vi "LS Acquisition Main (FPGA).vi"() -> ()   [LabVIEW 2013]
uses:
  <vilib>/rvi/Emulation/niFpgaSctlEmulationGetInTimedLoop.vi
  <vilib>/rvi/Emulation/niFpgaEmulationReportErrorSimple.vi
  <vilib>/rvi/Emulation/niFpgaGetClockAttributes.vi
  <vilib>/rvi/eio/common/nirviEmuTemplateMethod_errors.vi
  <vilib>/rvi/Emulation/niFpgaCriticalErrorInLSC.vi
  <vilib>/rvi/DataTransferAndStorage/Container/Common/niFpgaContainerExecOnDevCompGetState.vi
  <vilib>/rvi/FIFO/Fifo_Resource/nirvififoEmulationWriteFpgaImpl.vi
  <vilib>/rvi/DataTransferAndStorage/Container/Common/niFpgaContainerGetUniqueNameForEmu.vi
  <vilib>/rvi/interface/RandomDataEmulation/nirviRandomDataFPGAFIFO.vi
  <vilib>/rvi/interface/RandomDataEmulation/niFpgaRandomDataHandleErrors.vi
  <vilib>/rvi/eio/common/nirviEmuReportErrorAndStop.vi
  <vilib>/eio/EIONode/EIONode.xnode
  <vilib>/rvi/FXPMathLib/FxpAdd/XNode/nifxpmath_Add.xnode
  <vilib>/rvi/DataTransferAndStorage/Container/XNode/niFpgaContainer.xnode
  <vilib>/rvi/FIFO/Fifo_Resource/niFpgaFifoEmulationRefIn.vi
  <vilib>/rvi/FXPMathLib/sim/FxpSim.dll
panel:
  in  "B2offset":fxp<+/-,24,5>
  in  "B1offset":fxp<+/-,24,5>
  out "Anomaly Resamples":fxp<+/-,28,17>[](array[numeric])
  out "Bank2Active":bool
  out "Bank1Active":bool
  out "Bank2On":bool
  out "Bank1On":bool
  in  "Enable Readings":bool[](array[boolean])=[FALSE, FALSE, FALSE, FALSE, FALSE, FALSE, FALSE, FALSE, FALSE, FALSE, FALSE, FALSE]
  in  "Opens Resets":bool[](array[boolean])=[FALSE, FALSE, FALSE, FALSE, FALSE, FALSE, FALSE, FALSE, FALSE, FALSE]
  in  "Enable Opens":bool[](array[boolean])=[FALSE, FALSE, FALSE, FALSE, FALSE, FALSE, FALSE, FALSE, FALSE, FALSE]
  out "Opens Detected":u16[](array[numeric])
  out "Opens Loop Time (usec)":u32=1000
  in  "Bank2(Pulse/Const)":bool
  in  "Bank2Const(On/Off)":bool
  out "Cycle Starts":bool[](array[boolean])
  out "Cycles":u32[](array[numeric])
  in  "Bank1Const(On/Off)":bool
  in  "Bank1(Pulse/Const)":bool
  in  "PWM Period (Ticks)":u32=4000000
  in  "Duty (Ticks)":i32=2000000
  in  "Invert PWM?":bool=TRUE
  in  "Cycle Resets":bool[](array[boolean])=[FALSE, FALSE, FALSE, FALSE, FALSE, FALSE, FALSE, FALSE, FALSE, FALSE]
  in  "Points to Avg":i32=20
  in  "Enable Cycles":bool[](array[boolean])=[FALSE, FALSE, FALSE, FALSE, FALSE, FALSE, FALSE, FALSE, FALSE, FALSE]
  out "Total Cycles":u32[](array[numeric])
  in  "Cycle Threshold":fxp<+/-,28,17>=1.2001953125
  out "Analog Inputs":fxp<+/-,28,17>[](array[numeric])
  out "AI Loop Time (usec)":u32=70
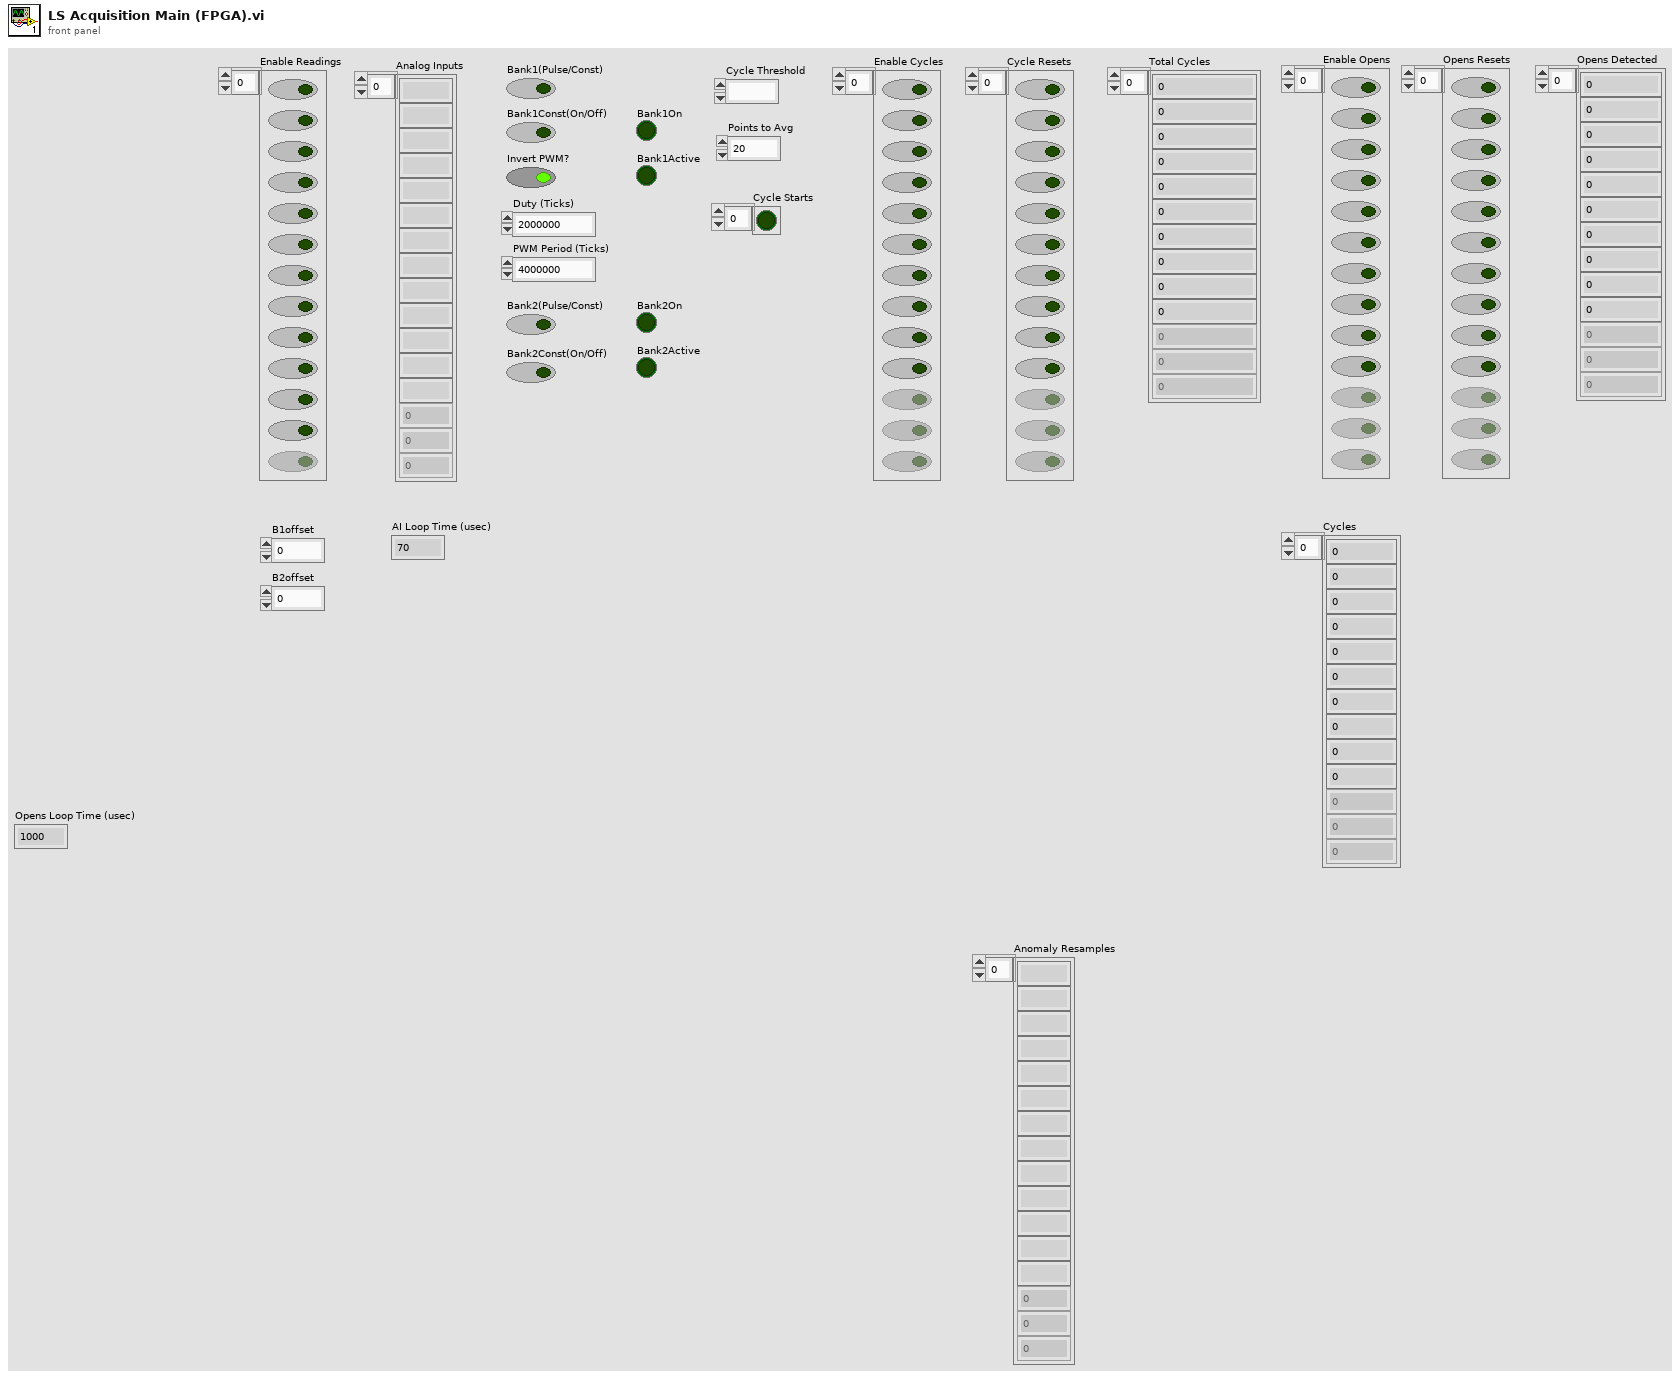
[diagram p1: front panel]
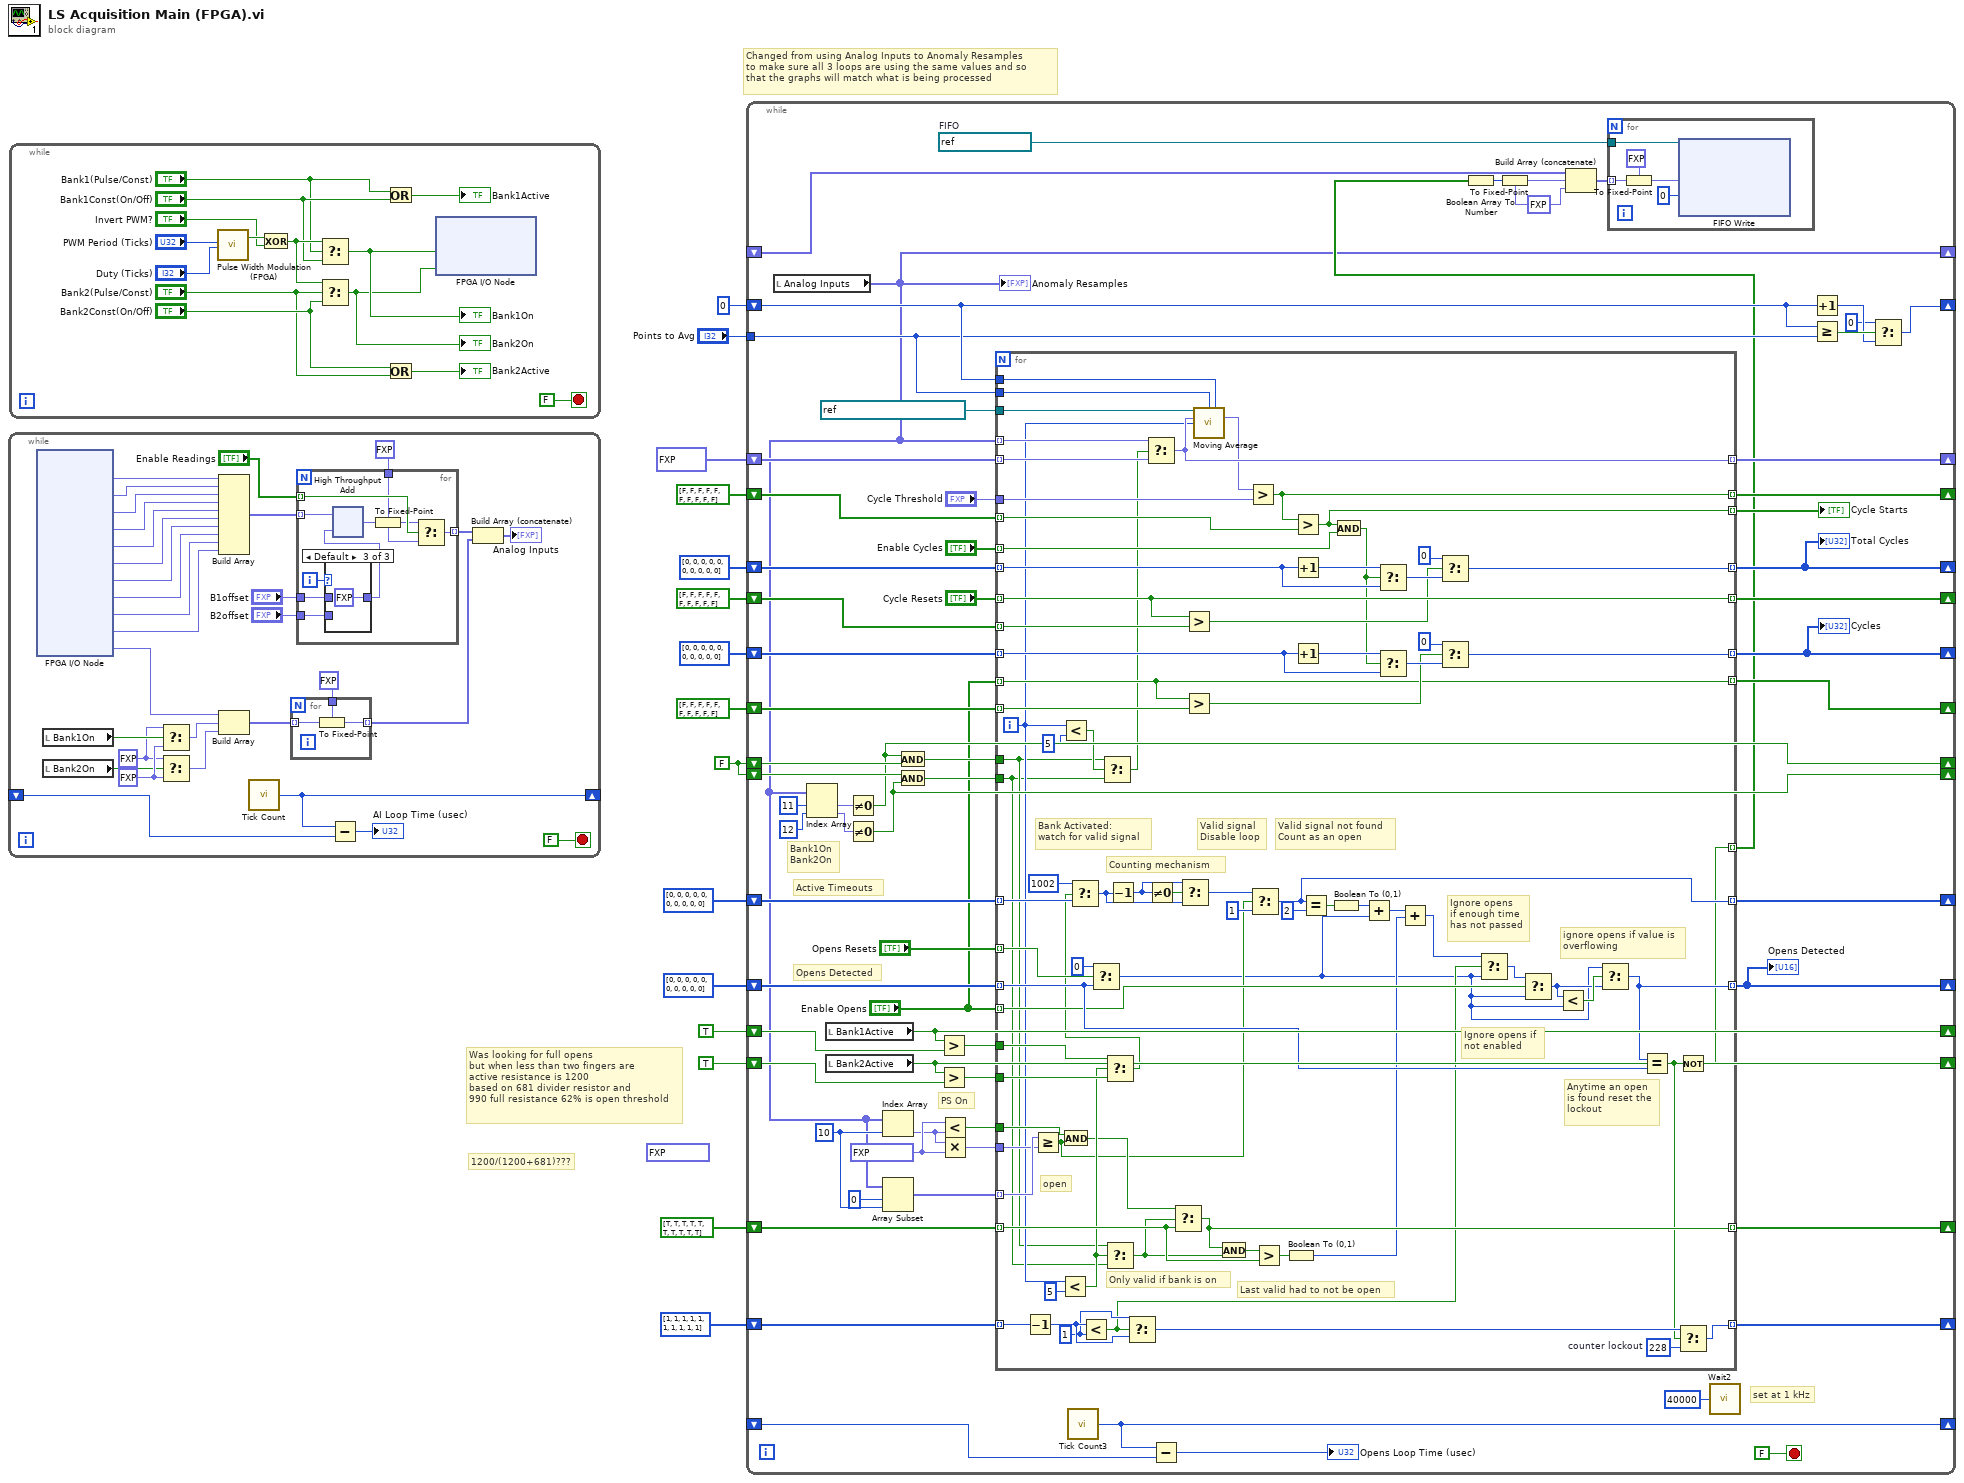
[diagram p0: block diagram]
diagram:
  (unwired) fxp<+,8,0> 0.94921875
  w7 = FALSE
  # "1200/(1200+681)???"
  # "Was looking for full opens\nbut when less than two fingers are\nactive resistance is 1200\nbased on 681 divider resistor and\n990 full resistance 62% is open threshold"
  # "Changed from using Analog Inputs to Anomaly Resamples\nto make sure all 3 loops are using the same values and so\nthat the graphs will match what is being processed"
  n1 = while {
    shift-right: [w45] -> _
    shift-left: _ -> [w44]
    stop <- FALSE stop-if-true
    w20 = fxp<+/-,24,5> 1.0 ("AI13")
    w23 = fxp<+/-,24,5> 0.0 ("AI13")
    n2 = xnode "FPGA I/O Node"() -> ("AI0"=w42:fxp<+/-,24,5>, "AI1"=w41:fxp<+/-,24,5>, "AI2"=w40:fxp<+/-,24,5>, "AI3"=w39:fxp<+/-,24,5>, "AI4"=w38:fxp<+/-,24,5>, "AI6"=w37:fxp<+/-,24,5>, "AI7"=w36:fxp<+/-,24,5>, "AI8"=w35:fxp<+/-,24,5>, "AI9"=w34:fxp<+/-,24,5>, "AI10"=w33:fxp<+/-,24,5>, "AI12"=w30:fxp<+/-,24,5>)  [unwired: 11 in, 11 out]
    n3 = local read "Bank1On"() -> (w22:bool)
    n4 = local read "Bank2On"() -> (w21:bool)
    n5 = Select(t=w20, s=w22, f=w23) -> (s? t:f=w19:fxp<+/-,24,5>)
    n6 = Select(t=w20, s=w21, f=w23) -> (s? t:f=w18:fxp<+/-,24,5>)
    n7 = Build Array(w42, w41, w40, w39, w38, w37, w36, w35, w34, w33) -> (w32:fxp<+/-,24,5>[])
    n8 = Build Array(w30, w19, w18) -> (w28:fxp<+/-,24,5>[])
    n9 = call "Tick Count"() -> ("Tick Count(uSec)"=w45:u32)
    n10 = for {
      tunnel: w28 -> [w49] mode=indexing
      tunnel: fxp<+/-,28,17> 0.0 ("AI0") -> [w48]
      tunnel: [w47] -> w27 mode=indexing
      n11 = To Fixed-Point(fixed-point type=w48, number=w49) -> (fixed-point=w47:fxp<+/-,28,17>)
    }
    n12 = for {
      tunnel: w32 -> [w52] mode=indexing
      tunnel: fxp<+/-,28,17> 0.0 ("AI0") -> [w57]
      tunnel: [w56] -> w26 mode=indexing
      tunnel: "Enable Readings" -> [w59] mode=indexing
      tunnel: "B1offset" -> [w54]
      tunnel: "B2offset" -> [w53]
      i -> [w55]
      n13 = case shown="Default" w55 {
        tunnel: w54 -> [w60 _ _]
        tunnel: w53 -> [_ w61 _]
        tunnel: [w60 w61 fxp<+/-,24,5> 0.0 ("B2offset")] -> w51
        frame 0..4 {
        }
        frame 5..9 {
        }
        frame Default {
        }
      }
      n14 = xnode "High Throughput Add"("x"=w52, "y"=w51) -> ("x+y"=w50:fxp<+/-,25,6>)
      n15 = To Fixed-Point(fixed-point type=w57, number=w50) -> (fixed-point=w58:fxp<+/-,28,17>)
      n16 = Select(t=w58, s=w59, f=w57) -> (s? t:f=w56:fxp<+/-,28,17>)
    }
    n17 = Subtract(x=w45, y=w44) -> (x-y=→"AI Loop Time (usec)":u32)
    n18 = Build Array (concatenate)(w26, w27) -> (→"Analog Inputs":fxp<+/-,28,17>[])
  }
  n19 = while {
    stop <- FALSE stop-if-true
    n20 = call "Pulse Width Modulation (FPGA).vi"("PWM Period (Ticks)"="PWM Period (Ticks)", "PWM Duty Cycle (Ticks)"="Duty (Ticks)") -> ("PWM DO"=w73:bool)  [unwired: 14 in, 3 out]
    n21 = Exclusive Or(1:"Invert PWM?", 2:w73) -> (0:w71:bool)
    n22 = Select(t=w71, s="Bank1(Pulse/Const)", f="Bank1Const(On/Off)") -> (s? t:f=w70:bool)
    "Bank1On" <- w70
    n23 = Select(t=w71, s="Bank2(Pulse/Const)", f="Bank2Const(On/Off)") -> (s? t:f=w69:bool)
    "Bank2On" <- w69
    n24 = Or(x="Bank1(Pulse/Const)", y="Bank1Const(On/Off)") -> (x .or. y?=→"Bank1Active":bool)
    n25 = Or(x="Bank2Const(On/Off)", y="Bank2(Pulse/Const)") -> (x .or. y?=→"Bank2Active":bool)
    n26 = xnode "FPGA I/O Node"("RMC/DIO0"=w70, "RMC/DIO1"=w69) -> ()  [unwired: 3 in, 3 out]
  }
  n27 = while {
    shift-right: [w143] -> _
    shift-left: _ -> [w142]
    shift-right: [w108] -> _
    shift-right: [w109] -> _
    shift-left: w7 -> [w138]
    shift-left: w7 -> [w139]
    tunnel: "Points to Avg" -> [w115]
    shift-right: [w134] -> _
    shift-left: 0 ("Moving Point Index") -> [w116]
    shift-right: [w117] -> _
    shift-left: fxp<+/-,28,17>[] [0.0, 0.0, 0.0, 0.0, 0.0, 0.0, 0.0, 0.0, 0.0, 0.0] ("Analog Inputs") -> [w119]
    shift-right: [w120] -> _
    shift-left: bool[] [FALSE, FALSE, FALSE, FALSE, FALSE, FALSE, FALSE, FALSE, FALSE, FALSE] -> [w122]
    shift-right: [w125] -> _
    shift-left: u32[] [0, 0, 0, 0, 0, 0, 0, 0, 0, 0] -> [w126]
    shift-right: [w127] -> _
    shift-left: bool[] [FALSE, FALSE, FALSE, FALSE, FALSE, FALSE, FALSE, FALSE, FALSE, FALSE] -> [w129]
    shift-right: [w131] -> _
    shift-left: u32[] [0, 0, 0, 0, 0, 0, 0, 0, 0, 0] -> [w132]
    shift-right: [w130] -> _
    shift-left: bool[] [FALSE, FALSE, FALSE, FALSE, FALSE, FALSE, FALSE, FALSE, FALSE, FALSE] -> [w133]
    shift-right: [w77] -> _
    shift-left: _ -> [w103]
    shift-right: [w96] -> _
    shift-left: u16[] [0, 0, 0, 0, 0, 0, 0, 0, 0, 0] -> [w100]
    shift-right: [w79] -> _
    shift-left: u8[] [0, 0, 0, 0, 0, 0, 0, 0, 0, 0] -> [w99]
    shift-right: [w85] -> _
    shift-left: TRUE ("Bank1Active") -> [w89]
    shift-right: [w84] -> _
    shift-left: TRUE ("Bank2Active") -> [w88]
    shift-right: [w95] -> _
    shift-left: bool[] [TRUE, TRUE, TRUE, TRUE, TRUE, TRUE, TRUE, TRUE, TRUE, TRUE] -> [w98]
    shift-right: [w94] -> _
    shift-left: u16[] [1, 1, 1, 1, 1, 1, 1, 1, 1, 1] -> [w97]
    stop <- FALSE stop-if-true
    w92 = fxp<+,8,0> 0.62109375
    w82 = 10 ("length")
    w104 = refnum<k21> "Analog Data"  # FIFO
    w106 = fxp<+/-,28,17> -15.0 ("AI0")
    # "PS On"
    # "Opens Detected"
    # "Active Timeouts"
    # "Bank1On\nBank2On"
    # "set at 1 kHz"
    n28 = local read "Analog Inputs"() -> (w77:fxp<+/-,28,17>[])
    "Anomaly Resamples" <- w77
    n29 = Index Array(array=w77, index #1=11 ("index"), index #2=12 ("index")) -> (element #1=w111:fxp<+/-,28,17>, element #2=w110:fxp<+/-,28,17>)
    n30 = local read "Bank1Active"() -> (w85:bool)
    n31 = local read "Bank2Active"() -> (w84:bool)
    n32 = Not Equal To 0?(x=w111) -> (x != 0?=w108:bool)
    n33 = Not Equal To 0?(x=w110) -> (x != 0?=w109:bool)
    n34 = Index Array(array=w77, index=w82) -> (element=w91:fxp<+/-,28,17>)
    n35 = Array Subset(array=w77, index=0, length=w82) -> (w83:fxp<+/-,28,17>[])
    n36 = And(x=w108, y=w139) -> (x .and. y?=w141:bool)
    n37 = And(x=w138, y=w109) -> (x .and. y?=w140:bool)
    n38 = Greater?(x=w85, y=w89) -> (0:w87:bool)
    n39 = Greater?(x=w84, y=w88) -> (0:w86:bool)
    n40 = Less?(x=w92, y=w91) -> (x < y?=w81:bool)
    n41 = Multiply(x=w91, y=w92) -> (x*y=w80:fxp<+/-,36,17>)
    n42 = for {
      tunnel: w141 -> [w154]
      tunnel: w140 -> [w153]
      tunnel: w133 -> [w231] mode=indexing
      tunnel: "Enable Opens" -> [w224] mode=indexing
      tunnel: w132 -> [w227] mode=indexing
      tunnel: [w226] -> w131 mode=indexing
      tunnel: [w224] -> w130 mode=indexing
      tunnel: w129 -> [w223] mode=indexing
      tunnel: "Cycle Resets" -> [w222] mode=indexing
      tunnel: [w222] -> w127 mode=indexing
      tunnel: w126 -> [w217] mode=indexing
      tunnel: [w216] -> w125 mode=indexing
      tunnel: "Enable Cycles" -> [w215] mode=indexing
      tunnel: "Cycle Threshold" -> [w212]
      tunnel: w122 -> [w213] mode=indexing
      tunnel: [w204] -> w121 mode=indexing
      tunnel: [w211] -> w120 mode=indexing
      tunnel: w119 -> [w210] mode=indexing
      tunnel: w77 -> [w201] mode=indexing
      tunnel: refnum<k21> "Running Avg Memory" ("Memory") -> [w209]
      tunnel: [w208] -> w117 mode=indexing
      tunnel: w116 -> [w207]
      tunnel: w115 -> [w206]
      tunnel: [w151] -> w102 mode=indexing
      tunnel: w100 -> [w200] mode=indexing
      tunnel: w99 -> [w199] mode=indexing
      tunnel: w98 -> [w198] mode=indexing
      tunnel: w97 -> [w197] mode=indexing
      tunnel: [w196] -> w96 mode=indexing
      tunnel: [w195] -> w95 mode=indexing
      tunnel: [w194] -> w94 mode=indexing
      tunnel: [w193] -> w79 mode=indexing
      tunnel: "Opens Resets" -> [w192] mode=indexing
      tunnel: "Enable Opens" -> [w191] mode=indexing
      tunnel: w87 -> [w190]
      tunnel: w86 -> [w189]
      tunnel: w83 -> [w188] mode=indexing
      tunnel: w81 -> [w187]
      tunnel: w80 -> [w186]
      i -> [w155]
      w160 = u16 228  # counter lockout
      w162 = u16 1 ("y")
      # "Ignore opens if\nnot enabled"
      # "Ignore opens\nif enough time\nhas not passed"
      # "Anytime an open\nis found reset the\nlockout"
      # "ignore opens if value is\noverflowing"
      # "Last valid had to not be open"
      # "Only valid if bank is on"
      # "open"
      # "Valid signal not found\nCount as an open"
      # "Valid signal\nDisable loop"
      # "Counting mechanism"
      # "Bank Activated:\nwatch for valid signal"
      n43 = Decrement(x=w197) -> (x-1=w163:u16)
      n44 = Greater Or Equal?(x=w188, y=w186) -> (x >= y?=w167:bool)
      n45 = Less?(x=w155, y=5) -> (x < y?=w184:bool)
      n46 = Less?(x=w155, y=5) -> (x < y?=w203:bool)
      n47 = And(x=w187, y=w167) -> (x .and. y?=w171:bool)
      n48 = Less?(x=w163, y=w162) -> (x < y?=w157:bool)
      n49 = Select(t=u16 0, s=w192, f=w199) -> (s? t:f=w156:u16)
      n50 = Select(t=w154, s=w203, f=w153) -> (s? t:f=w202:bool)
      n51 = Select(t=w190, s=w184, f=w189) -> (s? t:f=w172:bool)
      n52 = Select(t=u16 1002, s=w172, f=w200) -> (s? t:f=w173:u16)
      n53 = Select(t=w154, s=w184, f=w153) -> (s? t:f=w170:bool)
      n54 = Decrement(x=w173) -> (x-1=w177:u16)
      n55 = Select(t=w162, s=w157, f=w163) -> (s? t:f=w161:u16)
      n56 = Select(t=w201, s=w202, f=w210) -> (s? t:f=w208:fxp<+/-,28,17>)
      n57 = Not Equal To 0?(x=w177) -> (x != 0?=w176:bool)
      n58 = Select(t=w171, s=w170, f=w198) -> (s? t:f=w195:bool)
      n59 = Select(t=w177, s=w176, f=w173) -> (s? t:f=w178:u16)
      n60 = Greater?(x=w222, y=w223) -> (0:w218:bool)
      n61 = Greater?(x=w224, y=w231) -> (0:w225:bool)
      n62 = call "Moving Average.vi"("Memory In"=w209, "N (# of Ave Pts 127 max)"=w206, "Moving Point Index"=w207, "Data IN"=w208, "Channel#"=w155) -> ("Averaged Data"=w205:fxp<+/-,28,17>)  [unwired: 10 in]
      n63 = And(x=w195, y=w170) -> (x .and. y?=w166:bool)
      n64 = Greater?(x=w205, y=w212) -> (0:w211:bool)
      n65 = Select(t=w178, s=w167, f=u16 1) -> (s? t:f=w196:u16)
      n66 = Greater?(x=w166, y=w198) -> (0:w169:bool)
      n67 = Boolean To (0,1)(Boolean=w169) -> (0, 1=w168:i16)
      n68 = Greater?(x=w211, y=w213) -> (0:w204:bool)
      n69 = Increment(x=w217) -> (x+1=w219:u32)
      n70 = Increment(x=w227) -> (x+1=w230:u32)
      n71 = Equal?(x=w196, y=u16 2) -> (x = y?=w180:bool)
      n72 = Boolean To (0,1)(Boolean=w180) -> (0, 1=w181:i16)
      n73 = And(x=w204, y=w215) -> (x .and. y?=w214:bool)
      n74 = Add(x=w181, y=w156) -> (x+y=w182:u16)
      n75 = Select(t=w219, s=w214, f=w217) -> (s? t:f=w220:u32)
      n76 = Select(t=w230, s=w214, f=w227) -> (s? t:f=w229:u32)
      n77 = Add(x=w182, y=w168) -> (x+y=w158:u16)
      n78 = Select(t=u32 0, s=w218, f=w220) -> (s? t:f=w216:u32)
      n79 = Select(t=u32 0, s=w225, f=w229) -> (s? t:f=w226:u32)
      n80 = Select(t=w158, s=w157, f=w156) -> (s? t:f=w159:u16)
      n81 = Select(t=w159, s=w191, f=w156) -> (s? t:f=w164:u16)
      n82 = Less?(x=w164, y=w156) -> (x < y?=w165:bool)
      n83 = Select(t=w156, s=w165, f=w164) -> (s? t:f=w193:u16)
      n84 = Equal?(x=w193, y=w199) -> (x = y?=w152:bool)
      n85 = Not(x=w152) -> (.not. x?=w151:bool)
      n86 = Select(t=w161, s=w152, f=w160) -> (s? t:f=w194:u16)
    }
    "Total Cycles" <- w125
    "Cycles" <- w131
    "Cycle Starts" <- w121
    "Opens Detected" <- w79
    n87 = call "Tick Count3"() -> ("Tick Count(uSec)"=w143:u32)
    n88 = Subtract(x=w143, y=w142) -> (x-y=→"Opens Loop Time (usec)":u32)
    n89 = Boolean Array To Number(Boolean array=w102) -> (number=w107:u16)
    n90 = To Fixed-Point(fixed-point type=w106, number=w107) -> (fixed-point=w105:fxp<+/-,28,17>)
    n91 = Build Array (concatenate)(w103, w105, w106) -> (w114:fxp<+/-,28,17>[])
    n92 = for {
      tunnel: w104 -> [w150]
      tunnel: w114 -> [w149] mode=indexing
      n93 = To Fixed-Point(fixed-point type=fxp<+/-,22,11> 0.0 ("AI0"), number=w149) -> (fixed-point=w148:fxp<+/-,22,11>)
      n94 = xnode ("FIFO Write")("Element"=w148, "Timeout"=0, "FIFO In"=w150) -> ()  [unwired: 2 out]
    }
    n95 = call "Wait2"("Count(Ticks)"=u32 40000 ("Count(mSec)")) -> ()  [unwired: 1 out]
    n96 = Increment(x=w116) -> (x+1=w136:i32)
    n97 = Greater Or Equal?(x=w116, y=w115) -> (x >= y?=w137:bool)
    n98 = Select(t=0, s=w137, f=w136) -> (s? t:f=w134:i32)
  }
